vi "探头模板-28-32.vi"() -> ()   [LabVIEW 2017]
panel:
  in  "停止":bool=TRUE
  out "探头地址":T1(ring)
  out "探头信息":string
  out "探头状态":T2(ring)=enum."离线"
  in  "数据簇":T3
  out "测量值":dbl format="%.2g"
  out "单位":enum16{"μSv/h", "mSv/h"}(ring)
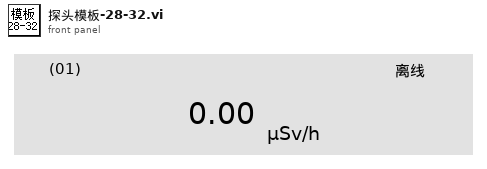
[diagram p1: front panel]
types:
  T1 = enum16{"(01)", "(02)", "(03)", "(04)", "(05)", "(06)", "(07)", "(08)", "(09)", "(10)", "(11)", "(12)", "(13)", "(14)", "(15)", "(16)", "(17)", "(18)", "(19)", "(20)", "(21)", "(22)", "(23)", "(24)", "(25)", "(26)", "(27)", "(28)", "(29)", "(30)", "(31)", "(32)", "(33)", "(34)", "(35)"}
  T2 = enum16{"正常", "未启用", "离线", "一级报警", "二级报警", "累积报警"}
  T3 = cluster{"启用状态？":bool, "测量值":cluster{"X":timestamp, "Y":dbl}, "限值簇":cluster{"限值1":dbl, "限值2":dbl, "探头限值":enum16{"一级限值", "二级限值"}}, "报警状态":enum16{"正常", "一级报警", "二级报警", "累积报警"}, "探头信息":string, "探头地址":i32, "累积剂量":cluster{"设备名称":string, "启用累积？":bool, "起始时间":timestamp, "累积剂量":dbl, "累积报警阈值":dbl}}
  T4 = cluster{"限值1":dbl, "限值2":dbl, "探头限值":enum16{"一级限值", "二级限值"}}
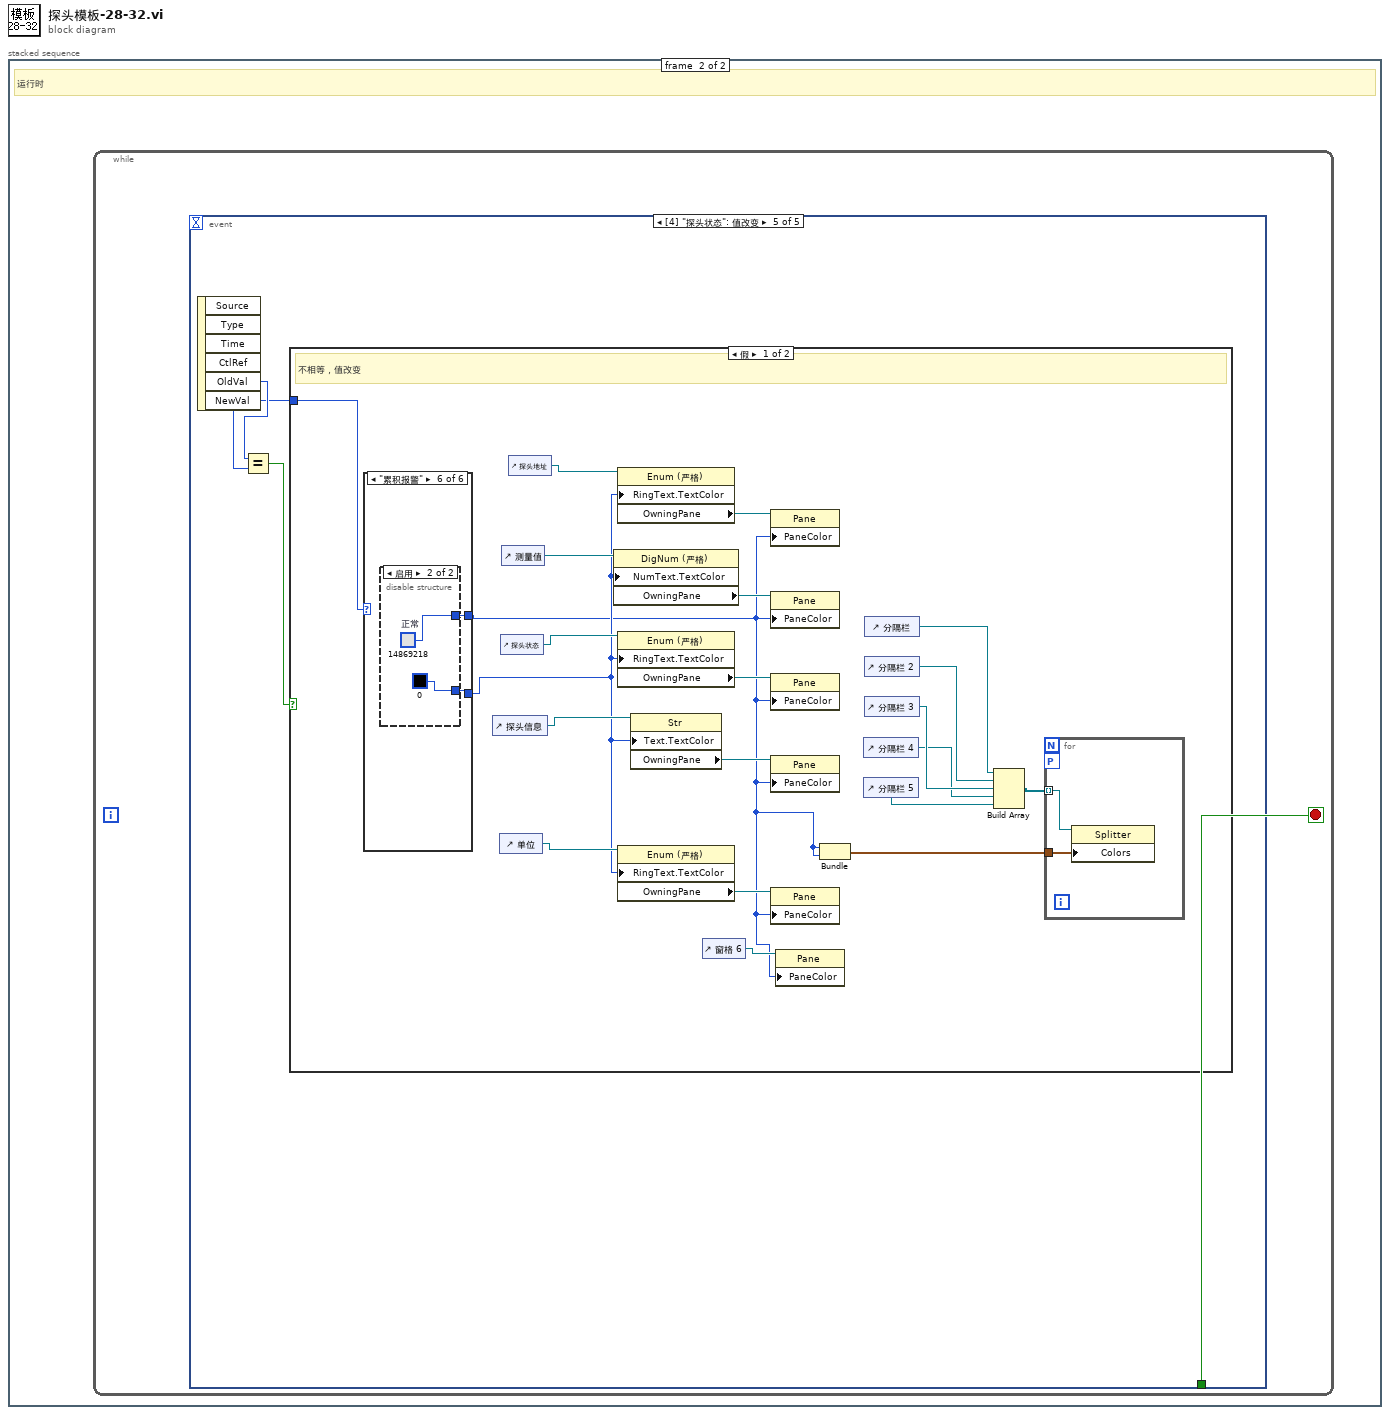
[diagram p0: block diagram]
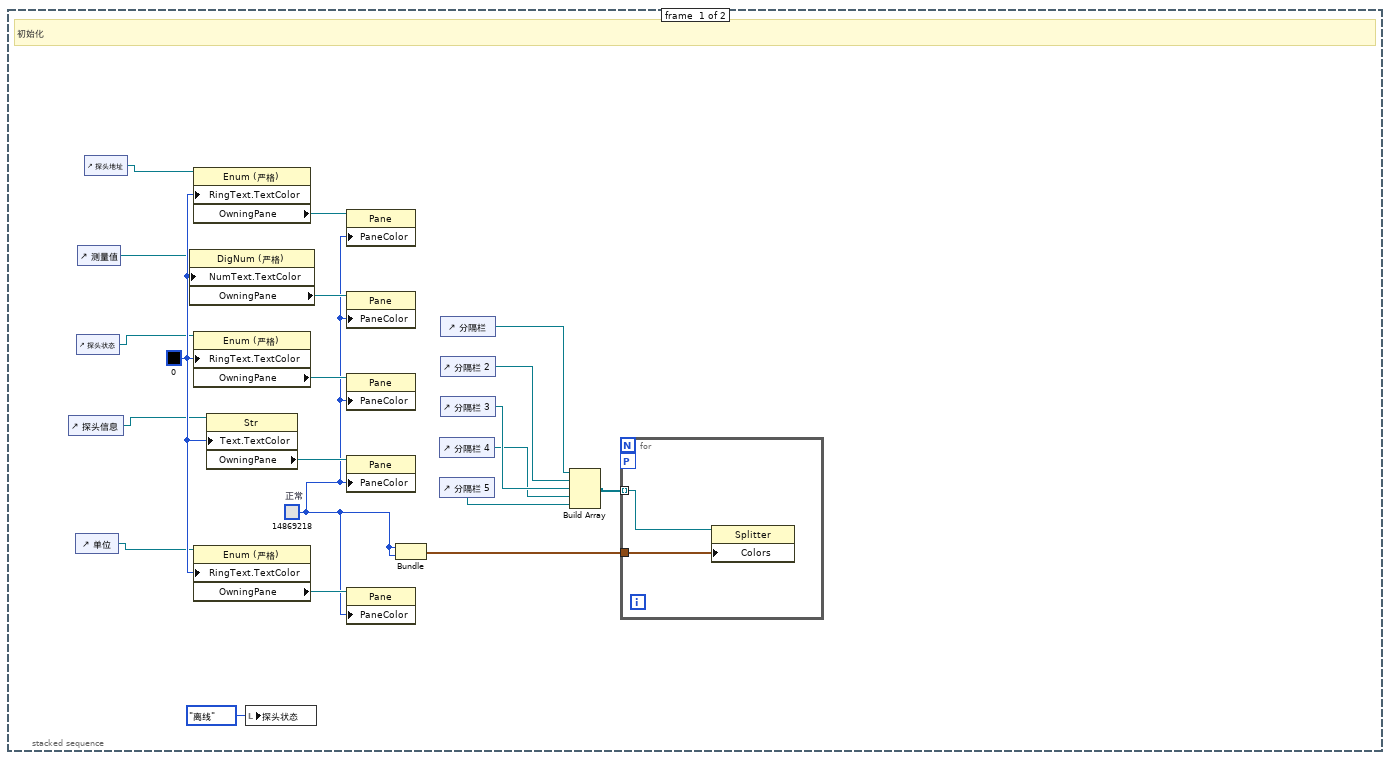
[diagram p2: hidden frame]
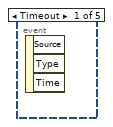
[diagram p3: hidden frame]
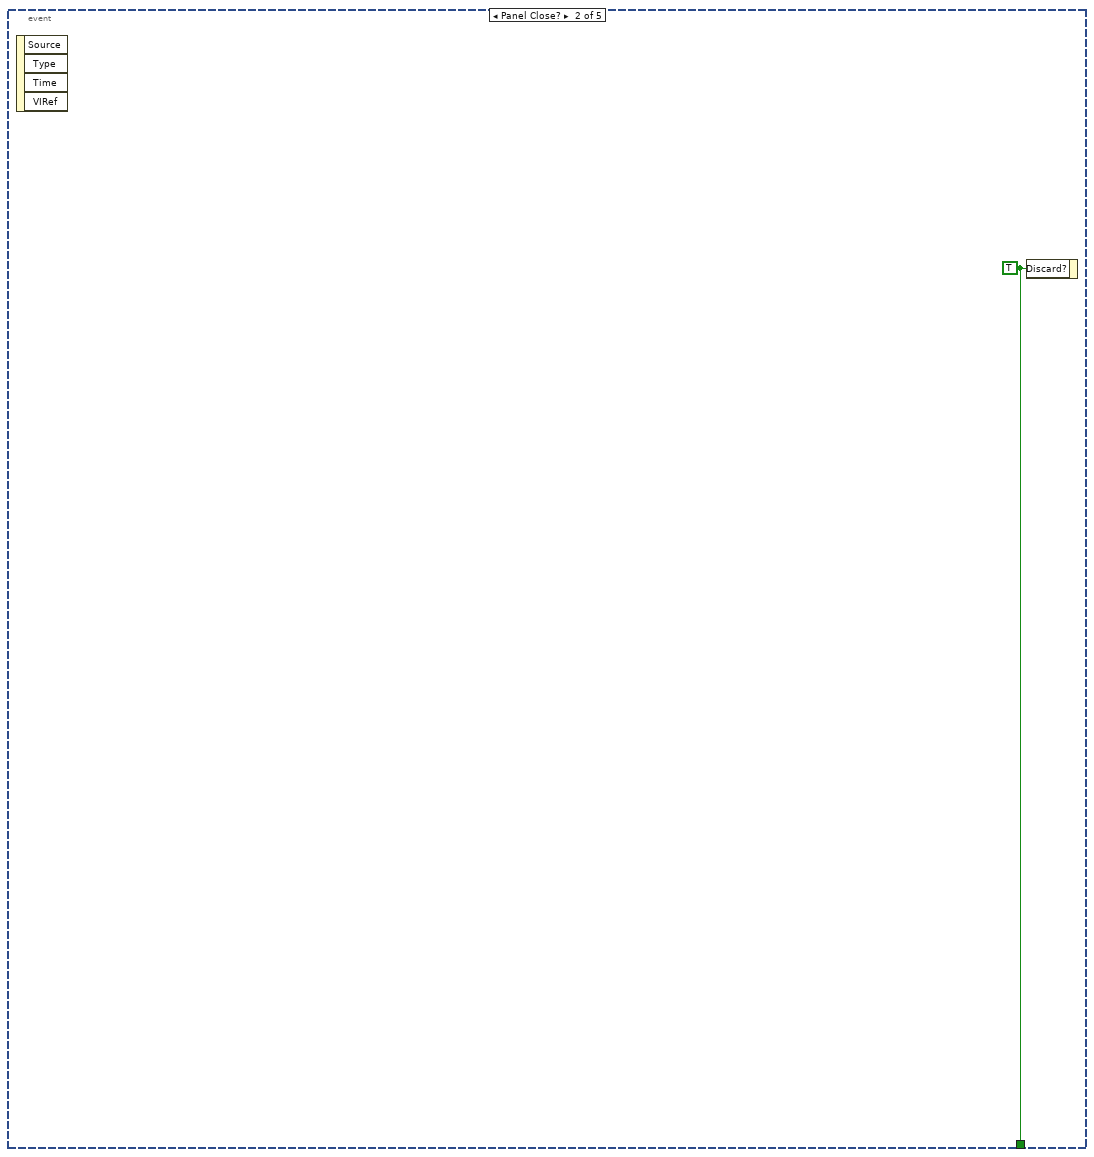
[diagram p4: hidden frame]
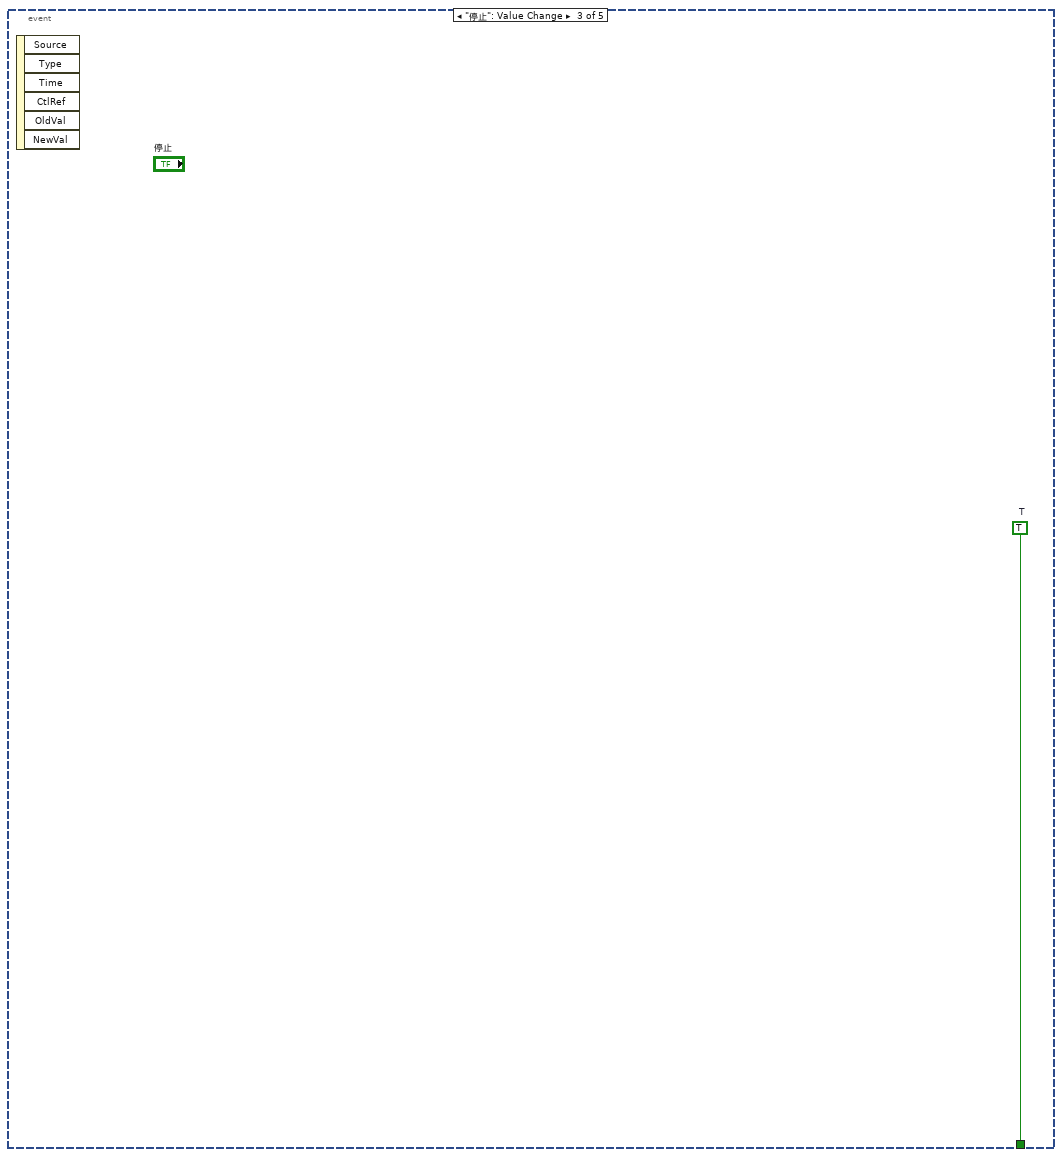
[diagram p5: hidden frame]
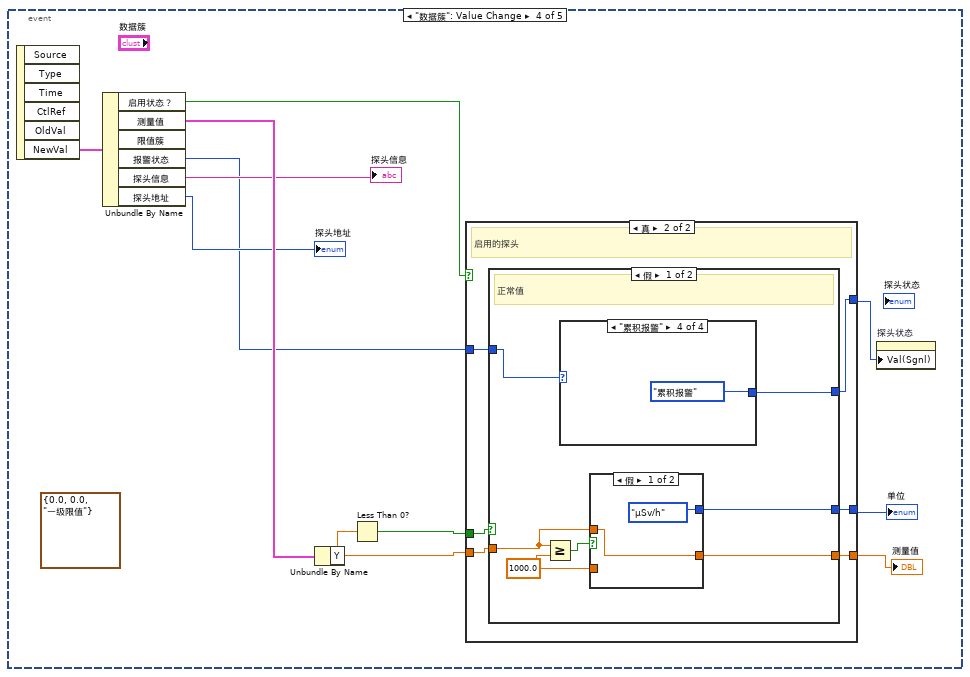
[diagram p6: hidden frame]
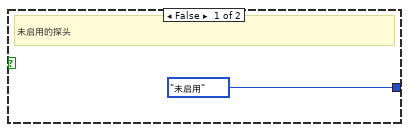
[diagram p7: hidden frame]
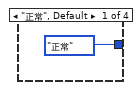
[diagram p8: hidden frame]
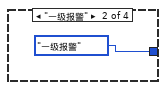
[diagram p9: hidden frame]
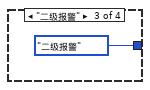
[diagram p10: hidden frame]
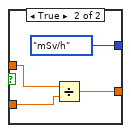
[diagram p11: hidden frame]
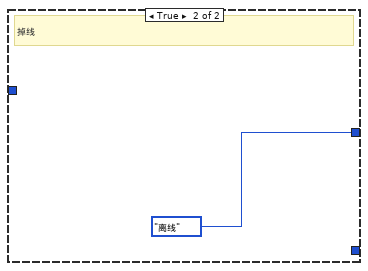
[diagram p12: hidden frame]
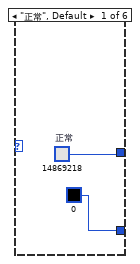
[diagram p13: hidden frame]
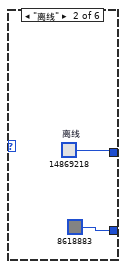
[diagram p14: hidden frame]
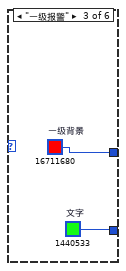
[diagram p15: hidden frame]
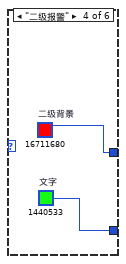
[diagram p16: hidden frame]
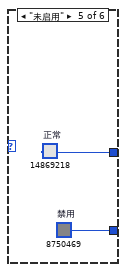
[diagram p17: hidden frame]
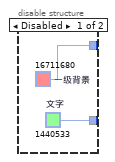
[diagram p18: hidden frame]
diagram:
  n1 = stacked-sequence {
    frame #0 {
      w15 = u32 0
      w13 = u32 14869218  # 正常
      # "初始化"
      n2 = control-ref of="探头信息"() -> (w2:refnum<vi>)
      n3 = control-ref of="单位"() -> (w1:refnum<vi>)
      n4 = control-ref of="探头状态"() -> (w3:refnum<vi>)
      n5 = control-ref of="测量值"() -> (w4:refnum<vi>)
      n6 = control-ref of="探头地址"() -> (w5:refnum<vi>)
      n7 = property on="属性节点" class="DigNum (严格)"(reference=w4, "NumText.TextColor"=w15) -> ("OwningPane"=w19:refnum<vi>)  [unwired: 1 in, 2 out]
      n8 = property on="属性节点" class="Enum (严格)"(reference=w5, "RingText.TextColor"=w15) -> ("OwningPane"=w20:refnum<vi>)  [unwired: 1 in, 2 out]
      n9 = property on="属性节点" class="Enum (严格)"(reference=w3, "RingText.TextColor"=w15) -> ("OwningPane"=w18:refnum<vi>)  [unwired: 1 in, 2 out]
      n10 = property on="属性节点" class="Enum (严格)"(reference=w1, "RingText.TextColor"=w15) -> ("OwningPane"=w16:refnum<vi>)  [unwired: 1 in, 2 out]
      n11 = property on="属性节点" class="Str"(reference=w2, "Text.TextColor"=w15) -> ("OwningPane"=w17:refnum<vi>)  [unwired: 1 in, 2 out]
      n12 = local write "探头状态"(enum16{"正常", "未启用", "离线", "一级报警", "二级报警"}."离线" ("探头状态")) -> ()
      n13 = property class="Pane"(reference=w20, "PaneColor"=w13) -> ()  [unwired: 1 in, 2 out]
      n14 = property class="Pane"(reference=w19, "PaneColor"=w13) -> ()  [unwired: 1 in, 2 out]
      n15 = property class="Pane"(reference=w18, "PaneColor"=w13) -> ()  [unwired: 1 in, 2 out]
      n16 = property class="Pane"(reference=w17, "PaneColor"=w13) -> ()  [unwired: 1 in, 2 out]
      n17 = property class="Pane"(reference=w16, "PaneColor"=w13) -> ()  [unwired: 1 in, 2 out]
      n18 = Bundle("正常"=w13, "正常"=w13) -> (w12:cluster{"正常":u32, "正常":u32})  [unwired: 1 in]
      n19 = control-ref of="分隔栏 4"() -> (w7:refnum<vi>)
      n20 = control-ref of="分隔栏 5"() -> (w6:refnum<vi>)
      n21 = control-ref of="分隔栏"() -> (w10:refnum<vi>)
      n22 = control-ref of="分隔栏 2"() -> (w9:refnum<vi>)
      n23 = control-ref of="分隔栏 3"() -> (w8:refnum<vi>)
      n24 = Build Array(w10, w9, w8, w7, w6) -> (w14:refnum<vi>[])
      n25 = for {
        tunnel: w12 -> [w22]
        workers-P: _ -> [_]
        tunnel: w14 -> [w21] mode=indexing
        n26 = property on="属性节点" class="Splitter"(reference=w21, "Colors"=w22) -> ()  [unwired: 1 in, 2 out]
      }
    }
    frame #1 {
      # "运行时"
      n27 = while {
        stop <- w23 stop-if-true
        n28 = event shown="[4] \"探头状态\": 值改变" {
          selector: _ -> [_ _ _ _ _]
          dyn-events: _ -> [_ _ _ _ _]
          timeout: _ -> [_ _ _ _ _]
          tunnel: [_ w24 w25 _ _] -> w23
          event Timeout {
            n29 = event-data() -> ()  [unwired: 1 in, 3 out]
          }
          event Panel Close? {
            w24 = TRUE ("放弃？")
            n30 = event-data() -> ()  [unwired: 1 in, 4 out]
            n31 = event-data("Discard?"=w24) -> ()  [unwired: 1 in, 1 out]
          }
          event "停止": Value Change {
            w25 = TRUE  # T
            n32 = event-data() -> ()  [unwired: 1 in, 6 out]
          }
          event "数据簇": Value Change {
            (unwired) T4 {"限值1"=0.0, "限值2"=0.0, "探头限值"=enum."一级限值"} ("探头限值簇")
            n33 = event-data() -> ("NewVal"=w31:T3)  [unwired: 1 in, 5 out]
            n34 = Unbundle By Name(w31) -> ("启用状态？"=w30:bool, "测量值"=w29:cluster{"X":timestamp, "Y":dbl}, "报警状态"=w26:enum16{"正常", "一级报警", "二级报警", "累积报警"}, "探头信息"=→"探头信息":string, "探头地址"=→"探头地址":i32)  [unwired: 1 out]
            n35 = Unbundle By Name(w29) -> ("Y"=w36:dbl)
            n36 = Less Than 0?(x=w36) -> (x < 0?=w35:bool)
            n37 = case shown="真" w30 {
              tunnel: w35 -> [_ w43]
              tunnel: w36 -> [_ w42]
              tunnel: [_ w41] -> w33
              tunnel: [_ w40] -> w34
              tunnel: [enum16{"正常", "未启用", "离线", "一级报警", "二级报警"}."未启用" ("探头状态") w39] -> w32
              tunnel: w26 -> [_ w38]
              frame False {
                # "未启用的探头"
              }
              frame True {
                # "启用的探头"
                n38 = case shown="假" w43 {
                  tunnel: w42 -> [w49 _]
                  tunnel: [w47 _] -> w41
                  tunnel: [w46 _] -> w40
                  tunnel: [w44 enum16{"正常", "未启用", "离线", "一级报警", "二级报警"}."离线" ("探头状态")] -> w39
                  tunnel: w38 -> [w45 _]
                  frame False {
                    w48 = 1000.0 ("y")
                    # "正常值"
                    n39 = Greater Or Equal?(x=w49, y=w48) -> (x >= y?=w50:bool)
                    n40 = case shown="\"累积报警\"" w45 {
                      tunnel: [enum16{"正常", "未启用", "离线", "一级报警", "二级报警"}."正常" ("探头状态") enum16{"正常", "未启用", "离线", "一级报警", "二级报警"}."一级报警" ("探头状态") enum16{"正常", "未启用", "离线", "一级报警", "二级报警"}."二级报警" ("探头状态") T2."累积报警" ("探头状态")] -> w44
                      frame "正常", Default {
                      }
                      frame "一级报警" {
                      }
                      frame "二级报警" {
                      }
                      frame "累积报警" {
                      }
                    }
                    n41 = case shown="假" w50 {
                      tunnel: w49 -> [w56 w60]
                      tunnel: w48 -> [_ w59]
                      tunnel: [w56 w58] -> w47
                      tunnel: [enum16{"μSv/h", "mSv/h"}."μSv/h" ("单位") enum16{"μSv/h", "mSv/h"}."mSv/h" ("单位")] -> w46
                      frame False {
                      }
                      frame True {
                        n42 = Divide(x=w60, y=w59) -> (x/y=w58:dbl)
                      }
                    }
                  }
                  frame True {
                    # "掉线"
                  }
                }
              }
            }
            "测量值" <- w33
            "单位" <- w34
            n43 = property on="探头状态" class="Enum (严格)"("Val(Sgnl)"=w32) -> ()  [unwired: 2 in, 2 out]
          }
          event "探头状态": Value Change {
            n44 = event-data() -> ("OldVal"=w64:T2, "NewVal"=w62:T2)  [unwired: 1 in, 4 out]
            n45 = Equal?(x=w64, y=w62) -> (x = y?=w63:bool)
            n46 = case shown="假" w63 {
              tunnel: w62 -> [w67 _]
              frame False {
                # "不相等，值改变"
                n47 = case shown="\"累积报警\"" w67 {
                  tunnel: [w86 w88 w91 w93 w94 w97] -> w65
                  tunnel: [u32 0 u32 8618883 w90 w92 w95 w96] -> w68
                  frame "正常", Default {
                    w86 = u32 14869218  # 正常
                  }
                  frame "离线" {
                    w88 = u32 14869218  # 离线
                  }
                  frame "一级报警" {
                    w90 = u32 1440533  # 文字
                    w91 = u32 16711680  # 一级背景
                  }
                  frame "二级报警" {
                    w92 = u32 1440533  # 文字
                    w93 = u32 16711680  # 二级背景
                  }
                  frame "未启用" {
                    w94 = u32 14869218  # 正常
                    w95 = u32 8750469  # 禁用
                  }
                  frame "累积报警" {
                    n48 = disable-structure shown="启用" {
                      disable-tunnel: [w99 w101] -> w97
                      disable-tunnel: [w98 u32 0] -> w96
                      frame Disabled {
                        w98 = u32 1440533  # 文字
                        w99 = u32 16711680  # 一级背景
                      }
                      frame Enabled {
                        w101 = u32 14869218  # 正常
                      }
                    }
                  }
                }
                n49 = control-ref of="探头信息"() -> (w70:refnum<vi>)
                n50 = control-ref of="单位"() -> (w69:refnum<vi>)
                n51 = control-ref of="探头状态"() -> (w71:refnum<vi>)
                n52 = control-ref of="测量值"() -> (w72:refnum<vi>)
                n53 = control-ref of="探头地址"() -> (w73:refnum<vi>)
                n54 = property on="属性节点" class="DigNum (严格)"(reference=w72, "NumText.TextColor"=w68) -> ("OwningPane"=w84:refnum<vi>)  [unwired: 1 in, 2 out]
                n55 = property on="属性节点" class="Enum (严格)"(reference=w73, "RingText.TextColor"=w68) -> ("OwningPane"=w85:refnum<vi>)  [unwired: 1 in, 2 out]
                n56 = property on="属性节点" class="Enum (严格)"(reference=w71, "RingText.TextColor"=w68) -> ("OwningPane"=w83:refnum<vi>)  [unwired: 1 in, 2 out]
                n57 = property on="属性节点" class="Enum (严格)"(reference=w69, "RingText.TextColor"=w68) -> ("OwningPane"=w81:refnum<vi>)  [unwired: 1 in, 2 out]
                n58 = property on="属性节点" class="Str"(reference=w70, "Text.TextColor"=w68) -> ("OwningPane"=w82:refnum<vi>)  [unwired: 1 in, 2 out]
                n59 = control-ref of="窗格 6"() -> (w66:refnum<vi>)
                n60 = property class="Pane"(reference=w85, "PaneColor"=w65) -> ()  [unwired: 1 in, 2 out]
                n61 = property class="Pane"(reference=w84, "PaneColor"=w65) -> ()  [unwired: 1 in, 2 out]
                n62 = property class="Pane"(reference=w83, "PaneColor"=w65) -> ()  [unwired: 1 in, 2 out]
                n63 = property class="Pane"(reference=w82, "PaneColor"=w65) -> ()  [unwired: 1 in, 2 out]
                n64 = property class="Pane"(reference=w81, "PaneColor"=w65) -> ()  [unwired: 1 in, 2 out]
                n65 = property class="Pane"(reference=w66, "PaneColor"=w65) -> ()  [unwired: 1 in, 2 out]
                n66 = Bundle("正常"=w65, "正常"=w65) -> (w79:cluster{"正常":u32, "正常":u32})  [unwired: 1 in]
                n67 = control-ref of="分隔栏 4"() -> (w75:refnum<vi>)
                n68 = control-ref of="分隔栏 5"() -> (w74:refnum<vi>)
                n69 = control-ref of="分隔栏"() -> (w78:refnum<vi>)
                n70 = control-ref of="分隔栏 2"() -> (w77:refnum<vi>)
                n71 = control-ref of="分隔栏 3"() -> (w76:refnum<vi>)
                n72 = Build Array(w78, w77, w76, w75, w74) -> (w80:refnum<vi>[])
                n73 = for {
                  tunnel: w79 -> [w103]
                  workers-P: _ -> [_]
                  tunnel: w80 -> [w102] mode=indexing
                  n74 = property on="属性节点" class="Splitter"(reference=w102, "Colors"=w103) -> ()  [unwired: 1 in, 2 out]
                }
              }
              frame True {
              }
            }
          }
        }
      }
    }
  }
